vi "Data Analyze.vi"(8 "error in (no error)":errorcluster caption="Error In", 9 "Identifier List":T1[](array[typedef]), 11 "Data":T2(c390)) -> (0 "error out":errorcluster caption="Error Out", 1 "Data Out":string[][](array[string]), 2 "Data":cluster{string, string, string}[](array[cluster]), 3 "Send Data":map{string, string}(c390))   [LabVIEW 2020]
uses:
  Global/Data Global/SDQ Data Type.ctl
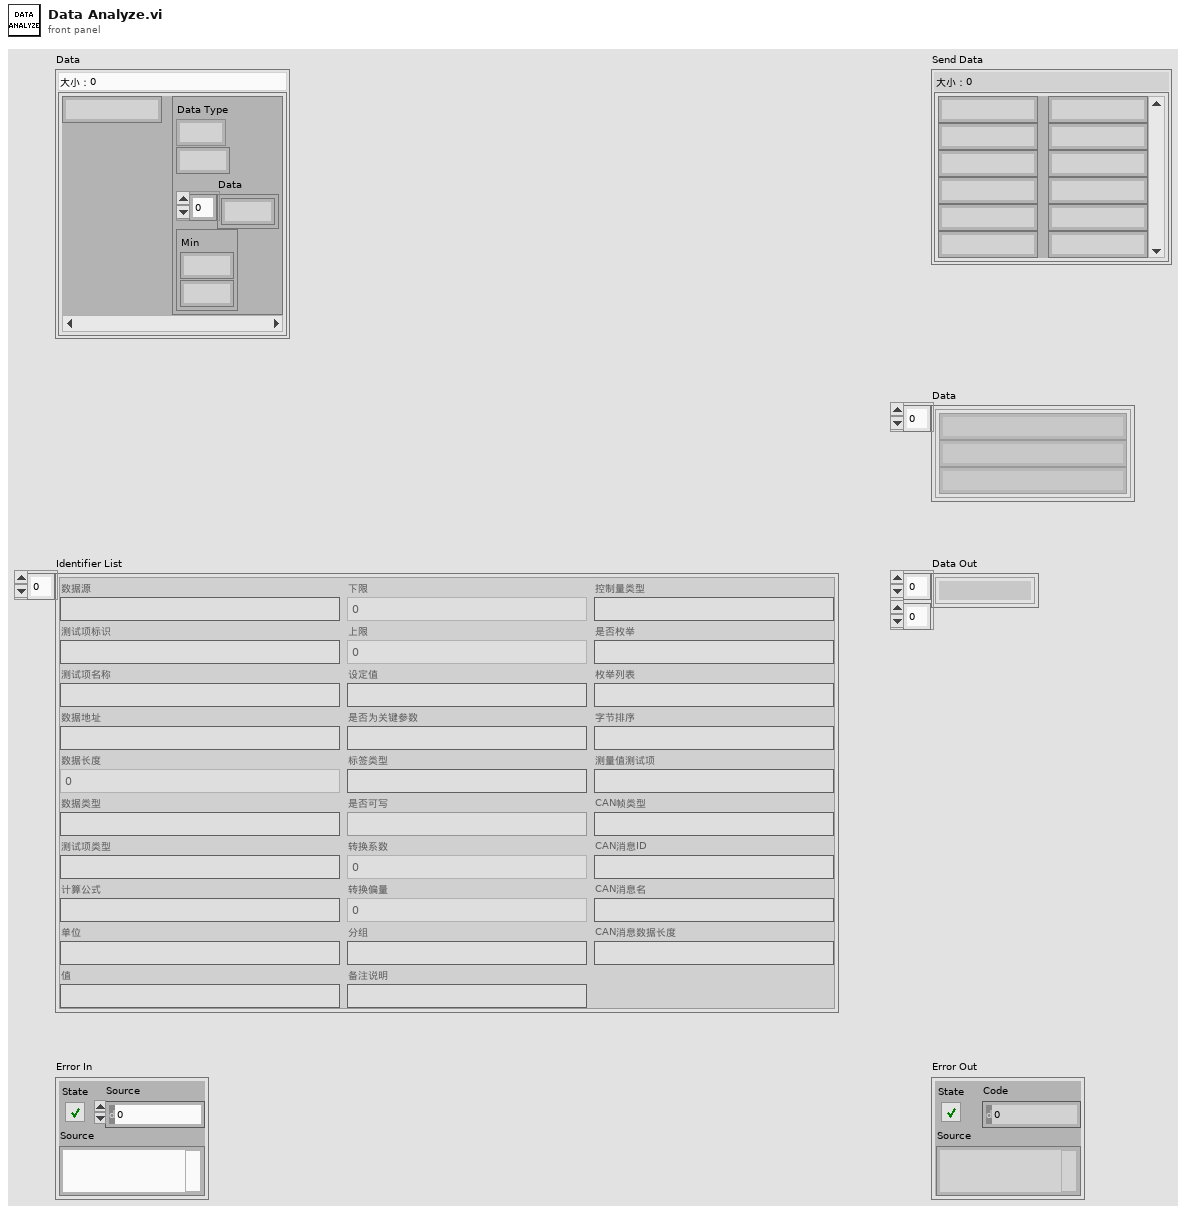
[diagram p1: front panel]
types:
  T1 = typedef "SDQ Data Type.ctl" = cluster{"CAN Length":string, "CAN Name":string, "CAN ID":string, "CAN Type":string, "Test Item":string, "Byte Order":string, "Instruction":string, "Control Type":string, "Group":string, "Offset":dbl, "Coefficient":dbl, "Write Enable":bool, "Lable Type":string, "Key?":string, "Set Value":string, "Upper":dbl, "Lower":dbl, "Unit":string, "Formula":string, "Test Item Type":string, "Length":i32, "Address":string, "Name":string, "Identifier":string, "Data Type":string, "Enumerate?":string, "Enumerate List":string, "Data":string, "Source":string}
  T2 = map{string, cluster{"Data Type":enum16{"I", "Q", "M", "D", "Count", "Timer"}, u16, "Data":u8[], cluster{"Min":u16, u16}}}
  T3 = cluster{"Data Type":enum16{"I", "Q", "M", "D", "Count", "Timer"}, u16, "Data":u8[], cluster{"Min":u16, u16}}
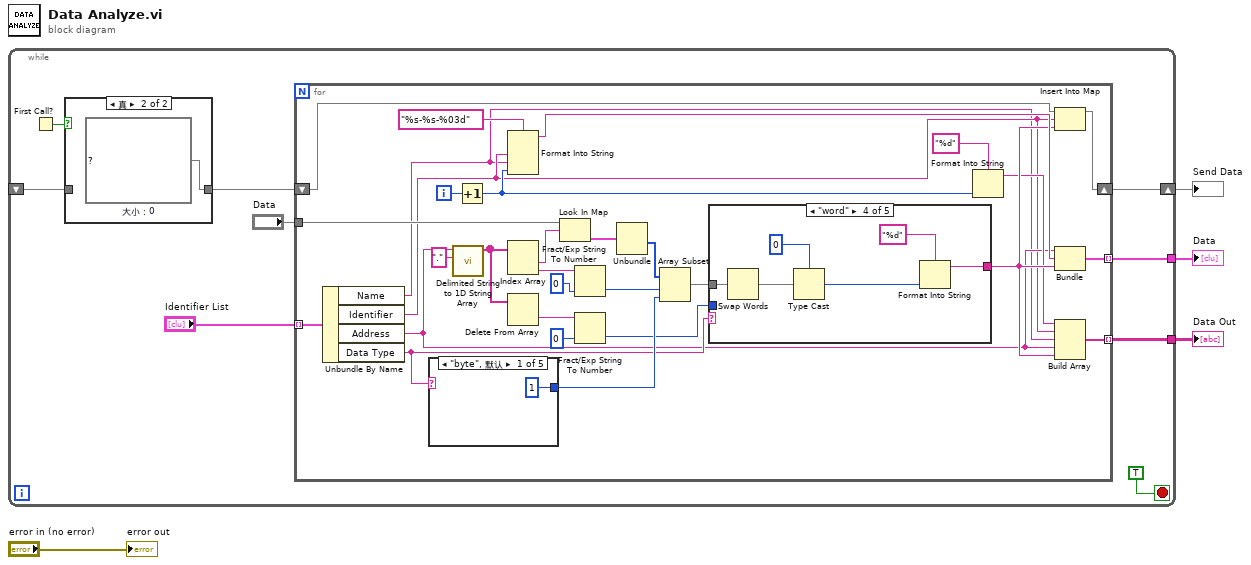
[diagram p0: block diagram]
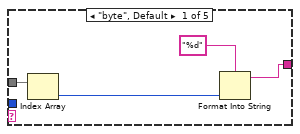
[diagram p3: hidden frame]
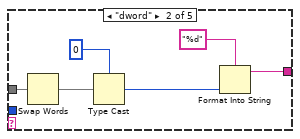
[diagram p4: hidden frame]
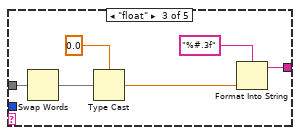
[diagram p5: hidden frame]
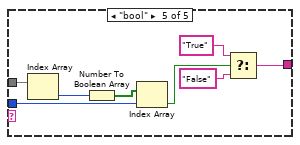
[diagram p6: hidden frame]
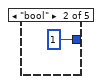
[diagram p7: hidden frame]
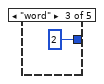
[diagram p8: hidden frame]
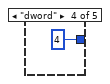
[diagram p9: hidden frame]
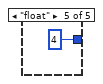
[diagram p10: hidden frame]
diagram:
  n1 = while {
    shift-right: [w9] -> w3
    shift-left: _ -> [w8]
    tunnel: [w7] -> w2
    tunnel: [w5] -> w1
    stop <- TRUE stop-if-true
    n2 = First Call?() -> (First Call?: T/F=w11:bool)
    n3 = case shown="真" w11 {
      tunnel: [w14 w15] -> w10
      tunnel: w8 -> [w14 _]
      frame False {
      }
      frame True {
        w15 = map{string, string} {}  # 大小：0
      }
    }
    n4 = for {
      tunnel: "Identifier List" -> [w45] mode=indexing
      tunnel: "Data" -> [w43]
      shift-right: [w29] -> w9
      shift-left: w10 -> [w30]
      tunnel: [w25] -> w7 mode=indexing
      tunnel: [w24] -> w5 mode=indexing
      i -> [w26]
      n5 = Unbundle By Name(w45) -> ("Name"=w16:string, "Identifier"=w17:string, "Address"=w18:string, "Data Type"=w33:string)
      n6 = case shown="\"byte\", 默认" w33 {
        tunnel: [1 1 2 4 4] -> w34
        frame "byte", Default {
        }
        frame "bool" {
        }
        frame "word" {
        }
        frame "dword" {
        }
        frame "float" {
        }
      }
      n7 = call <vilib>:"Delimited String to 1D String Array.vi"("delimiter"=".", "delimited string"=w18) -> ("string array"=w40:string[])  [unwired: 9 in]
      n8 = Increment(x=w26) -> (x+1=w20:i32)
      n9 = Format Into String(format string="%s-%s-%03d" ("格式字符串"), w17, w16, w20) -> (resulting string=w23:string)  [unwired: 2 in, 1 out]
      n10 = Index Array(array=w40) -> (element #1=w42:string, element #2=w36:string)  [unwired: 2 in]
      n11 = Delete From Array(array=w40) -> (deleted portion=w38:string)  [unwired: 2 in, 1 out]
      n12 = Look In Map(map=w43, key=w42) -> (value=w41:T3)  [unwired: 1 in, 1 out]
      n13 = Fract/Exp String To Number(string=w36, default (0 dbl)=0 ("默认(0 DBL)")) -> (number=w35:i32)  [unwired: 2 in, 1 out]
      n14 = Fract/Exp String To Number(string=w38, default (0 dbl)=0 ("默认(0 DBL)")) -> (number=w32:i32)  [unwired: 2 in, 1 out]
      n15 = Unbundle(w41) -> ("Data"=w28:u8[])  [unwired: 3 out]
      n16 = Array Subset(array=w28, index=w35, length=w34) -> (w31:u8[])
      n17 = case shown="\"word\"" w33 {
        tunnel: w32 -> [_ _ _ _ w72]
        tunnel: w31 -> [w49 w51 w59 w63 w75]
        tunnel: [w46 w54 w60 w66 w68] -> w22
        frame "byte", Default {
          n18 = Index Array(array=w49) -> (element=w47:u8)  [unwired: 1 in]
          n19 = Format Into String(format string="%d" ("格式字符串"), w47) -> (resulting string=w46:string)  [unwired: 2 in, 1 out]
        }
        frame "dword" {
          n20 = Swap Words(1:w51) -> (0:w50:u8[])
          n21 = Type Cast(type=u32 0, x=w50) -> (*(type *) &x=w52:u32)
          n22 = Format Into String(format string="%d" ("格式字符串"), w52) -> (resulting string=w54:string)  [unwired: 2 in, 1 out]
        }
        frame "float" {
          n23 = Swap Words(1:w59) -> (0:w56:u8[])
          n24 = Type Cast(type=sgl 0.0, x=w56) -> (*(type *) &x=w57:sgl)
          n25 = Format Into String(format string="%#.3f" ("格式字符串"), w57) -> (resulting string=w60:string)  [unwired: 2 in, 1 out]
        }
        frame "word" {
          n26 = Swap Words(1:w63) -> (0:w62:u8[])
          n27 = Type Cast(type=u16 0, x=w62) -> (*(type *) &x=w64:u16)
          n28 = Format Into String(format string="%d" ("格式字符串"), w64) -> (resulting string=w66:string)  [unwired: 2 in, 1 out]
        }
        frame "bool" {
          n29 = Index Array(array=w75) -> (element=w74:u8)  [unwired: 1 in]
          n30 = Number To Boolean Array(number=w74) -> (Boolean array=w73:bool[])
          n31 = Index Array(array=w73, index=w72) -> (element=w71:bool)
          n32 = Select(t="True", s=w71, f="False") -> (s? t:f=w68:string)
        }
      }
      n33 = Format Into String(format string="%d" ("格式字符串"), w20) -> (resulting string=w19:string)  [unwired: 2 in, 1 out]
      n34 = Insert Into Map(map in=w30, key=w17, value=w22) -> (map out=w29:map{string, string})  [unwired: 2 out]
      n35 = Bundle("Address"=w18, w23, w22) -> (w25:cluster{"Address":string, string, string})  [unwired: 1 in]
      n36 = Build Array(w19, w17, w16, w18, w22) -> (w24:string[])
    }
  }
  "Send Data" <- w3
  "Data" <- w2
  "Data Out" <- w1
  "error out" <- "error in (no error)"
